vi "WriteTree.vi"(8 "error in":errorcluster, 11 "CEF_Hierachy repository in":refnum<class "CEF_HierarchyRepo.lvclass">) -> (0 "error out":errorcluster, 2 "root":T1, 3 "repository out":refnum<class "CEF_Repository.lvclass">)   [LabVIEW 2025, in "CEF.lvlib" / "CEF_HierarchyRepo.lvclass"]
doc: "Transfers information between the repo and the tree control. This method should be called after the custom views are called or saving to disk.Copyright 2017 National Instruments Corporation\n\nLicensed under the Apache License, Version 2.0 (the \"License\"); you may not use this file except in compliance with the License. You may obtain a copy of the License at http://www.apache.org/licenses/LICENSE-2.0\nUnless required by applicable law or agreed to in writing, software distributed under the License is distributed on an \"AS IS\" BASIS, WITHOUT WARRANTIES OR CONDITIONS OF ANY KIND, either express or implied. See the License for the specific language governing permissions and limitations under the License."
uses:
  CEF_HierarchyRepo.lvclass
  C:/Working copy/tss/Plugin/CEF/Repository/CEF_Repository.lvclass
  Repository/CEF_Repository.lvclass
  Node/NodeRef.ctl
  Node/CEF_Node.lvclass
  Node/FromRepoCluster.ctl
  CEF_HierarchyRepo.lvclass/CEF_HierarchyRepo.ctl
  serializable node/CEF_serializable node.lvclass
  CEF.lvlib
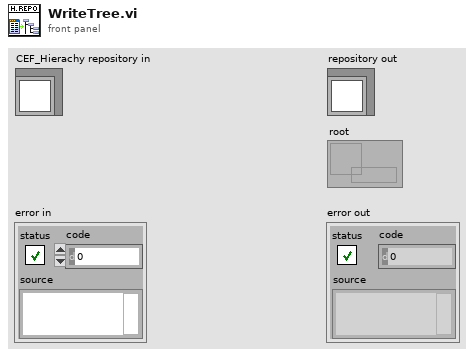
[diagram p1: front panel]
types:
  T1 = typedef "CEF.lvlib/CEF_Node.lvclass/NodeRef.ctl" = refnum<data-value>
  T2 = typedef "CEF.lvlib/CEF_Node.lvclass/FromRepoCluster.ctl" = cluster{"tag":string, "tags":string[], "classes":string[], "index":i32, "variant":variant}
  T3 = typedef "CEF.lvlib/CEF_HierarchyRepo.lvclass/memory hierarchy.ctl" = cluster{"hierarchy structure":T4, "instance data":refnum<class "CEF_serializable configuration.lvclass">[]}
  T4 = typedef "CEF.lvlib/CEF_HierarchyRepo.lvclass/full hierarchy.ctl" = cluster{"root":string, "hierarchy":T5[]}
  T5 = typedef "CEF.lvlib/hierarchy element.ctl" = cluster{"current node":string, "children":string[]}
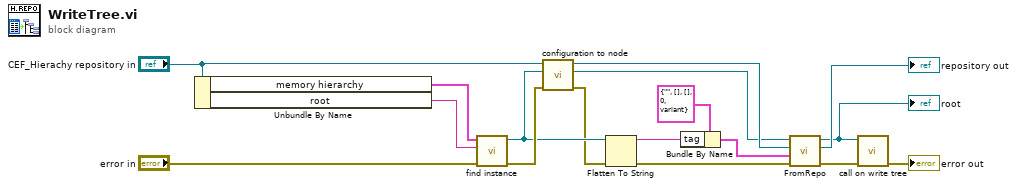
[diagram p0: block diagram]
diagram:
  n1 = Unbundle By Name("CEF_Hierachy repository in") -> ("memory hierarchy"=w14:T3, "root"=w16:string)
  n2 = call "find instance.vi"("error in"="error in", "ID"=w16, "memory hierarchy"=w14) -> ("error out"=w10:errorcluster, "CEF_Serialize configuration"=w6:refnum<class "CEF_serializable configuration.lvclass">)  [unwired: 7 in]
  n3 = call-dynamic "configuration to node.vi"("error in"=w10, "CEF_Configuration"=w6, "CEF_Hierarchy repo in"="CEF_Hierachy repository in") -> ("error out"=w1:errorcluster, "CEF_Serialize node"=w11:refnum<class "CEF_serializable node.lvclass">, "CEF_Hierarchy repo out"=w12:refnum<class "CEF_HierarchyRepo.lvclass">)  [unwired: 6 in]
  n4 = Flatten To String(anything=w6, error in (no error)=w1) -> (data string=w5:string, error out=w7:errorcluster)  [unwired: 2 in, 1 out]
  n5 = Bundle By Name(cluster=T2 {"tag"="", "tags"=[], "classes"=[], "index"=0, "variant"=variant} ("from repo cluster"), "tag"=w5) -> (w8:T2)
  n6 = call-dynamic "FromRepo.vi"("error in"=w7, "from repo cluster"=w8, "repository in"=w12, "CEF_configuration"=w11) -> ("error out"=w4:errorcluster, "repository out"=→"repository out":refnum<class "CEF_Repository.lvclass">, "node"=w2:T1)  [unwired: 5 in]
  "root" <- w2
  n7 = call "call on write tree.vi"("error in"=w4, "root"=w2) -> ("error out"=→"error out":errorcluster)  [unwired: 9 in]
